vi "Ball Velocity.vi"(11 "Ball":T1) -> (3 "Velocity":dbl[](array[numeric]))   [LabVIEW 2016]
uses:
  Core/AI Ball.ctl
panel:
  in  "Boolean":bool
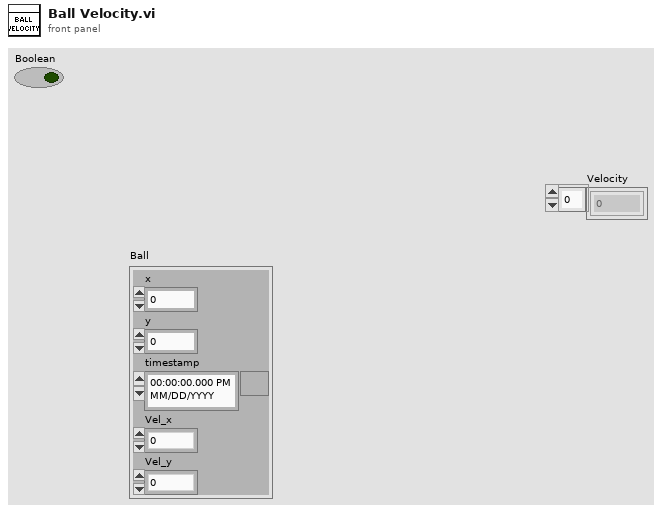
[diagram p1: front panel]
types:
  T1 = typedef "AI Ball.ctl" = cluster{"x":dbl, "y":dbl, "timestamp":timestamp, "Vel_x":dbl, "Vel_y":dbl}
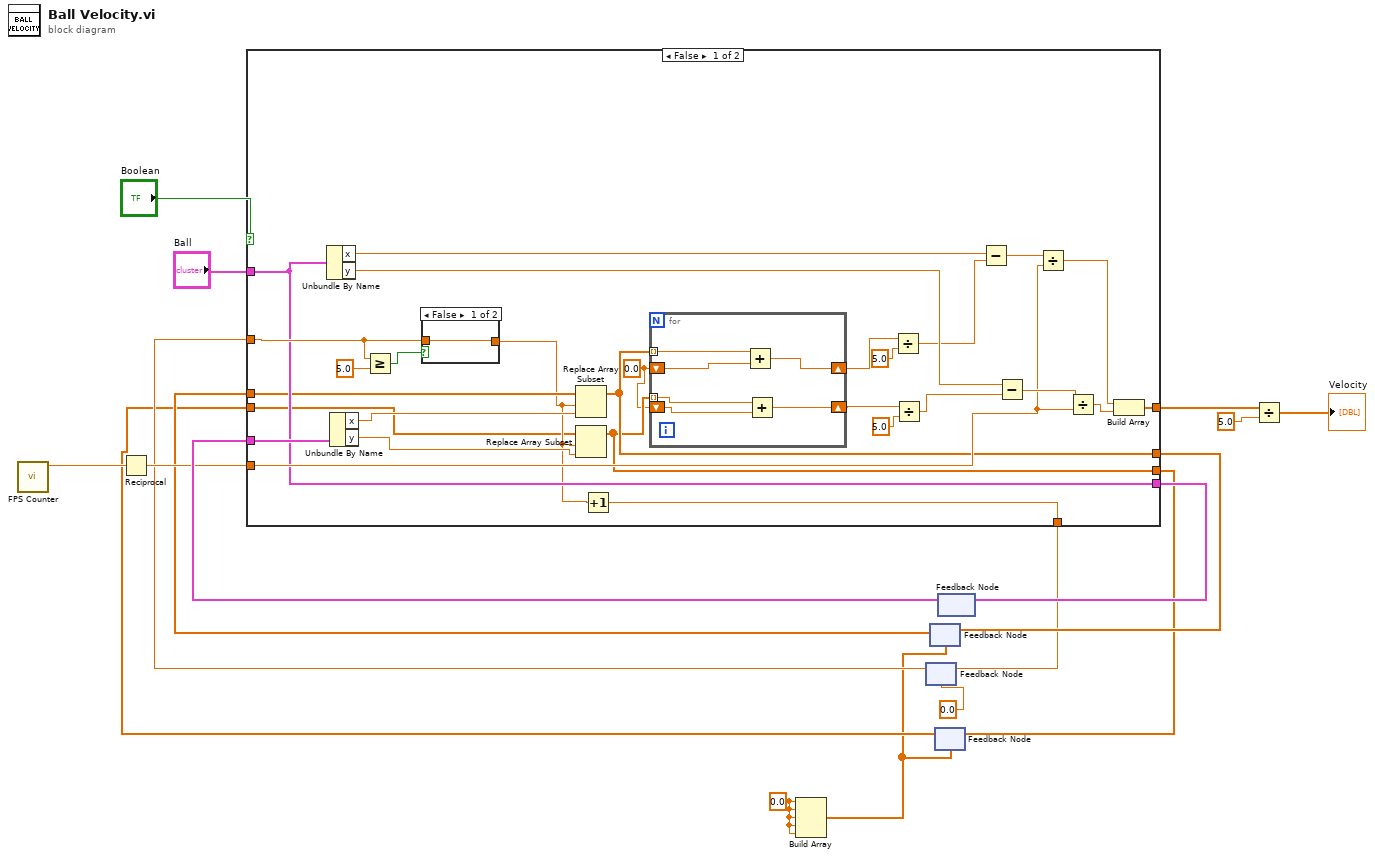
[diagram p0: block diagram]
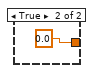
[diagram p2: hidden frame]
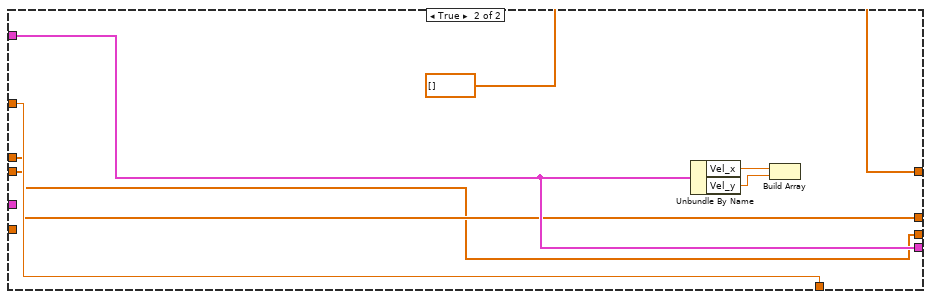
[diagram p3: hidden frame]
diagram:
  w5 = 0.0 ("element")
  n1 = call "FPS Counter.vi"() -> ("Numeric"=w14:dbl)  [unwired: 11 in]
  n2 = Reciprocal(x=w14) -> (1/x=w13:dbl)
  n3 = Build Array(w5, w5, w5, w5, w5) -> (w4:dbl[])
  n4 = feedback #1(0.0) -> (w9:dbl)
  n5 = feedback #2(w4) -> (w12:dbl[])
  n6 = feedback #3(w4) -> (w6:dbl[])
  n7 = feedback #4() -> (w16:T1)  [unwired: 1 in]
  n8 = case shown="False" "Boolean" {
    tunnel: "Ball" -> [w33 w58]
    tunnel: [w41 dbl[] [] ("Velocity")] -> w3
    tunnel: [w33 w58] -> w17
    tunnel: w16 -> [w46 _]
    tunnel: w13 -> [w38 _]
    tunnel: w12 -> [w28 w56]
    tunnel: [w32 w56] -> w11
    tunnel: [w37 w57] -> w10
    tunnel: w9 -> [w35 w57]
    tunnel: [w21 w55] -> w7
    tunnel: w6 -> [w20 w55]
    frame False {
      w19 = 0.0
      n9 = Unbundle By Name(w33) -> ("x"=w45:dbl, "y"=w44:dbl)
      n10 = Unbundle By Name(w46) -> ("x"=w29:dbl, "y"=w27:dbl)
      n11 = Greater Or Equal?(x=w35, y=5.0) -> (x >= y?=w36:bool)
      n12 = case shown="False" w36 {
        tunnel: w35 -> [w53 _]
        tunnel: [w53 0.0] -> w26
        frame False {
        }
        frame True {
        }
      }
      n13 = Replace Array Subset(array=w28, new element=w29, index=w26) -> (w32:dbl[])
      n14 = Replace Array Subset(array=w20, new element=w27, index=w26) -> (w21:dbl[])
      n15 = Increment(x=w26) -> (x+1=w37:dbl)
      n16 = for {
        tunnel: w32 -> [w52] mode=indexing
        shift-right: [w50] -> w31
        shift-left: w19 -> [w51]
        tunnel: w21 -> [w47] mode=indexing
        shift-right: [w49] -> w23
        shift-left: w19 -> [w48]
        n17 = Add(x=w52, y=w51) -> (x+y=w50:dbl)
        n18 = Add(x=w47, y=w48) -> (x+y=w49:dbl)
      }
      n19 = Divide(x=w31, y=5.0) -> (x/y=w25:dbl)
      n20 = Divide(x=w23, y=5.0) -> (x/y=w22:dbl)
      n21 = Subtract(x=w45, y=w25) -> (x-y=w43:dbl)
      n22 = Subtract(x=w44, y=w22) -> (x-y=w42:dbl)
      n23 = Divide(x=w43, y=w38) -> (x/y=w40:dbl)
      n24 = Divide(x=w42, y=w38) -> (x/y=w39:dbl)
      n25 = Build Array(w40, w39) -> (w41:dbl[])
    }
    frame True {
      n26 = Unbundle By Name(w58) -> ("Vel_x"=w61:dbl, "Vel_y"=w60:dbl)
      n27 = Build Array(w61, w60) -> ()  [unwired: 1 out]
    }
  }
  n28 = feedback-in #1(w10) -> ()
  n29 = feedback-in #2(w11) -> ()
  n30 = feedback-in #3(w7) -> ()
  n31 = feedback-in #4(w17) -> ()
  n32 = Divide(x=w3, y=5.0) -> (x/y=→"Velocity":dbl[])
